vi "PC_AO to DCCM no trigger_Current.vi"() -> ()   [LabVIEW 2021]
uses:
  DC-RMS Current Measurement/Typedefs/Range and Terminal Settings.ctl
  DC-RMS Current Measurement/Typedefs/Specific Channel Settings.ctl
  DC-RMS Current Measurement/Typedefs/DC and RMS Current Measurements.ctl
  DC Voltage Generation/DAQ_DC Voltage Generation.lvlib
  DC-RMS Current Measurement/DAQ_DC-RMS Current Measurement.lvlib
panel:
  out "Current Waveforms":waveform(dbl)[](graph)=[{"t0"=timestamp(3825152084.7836895 s since 1904-01-01), "dt"=9.999999999999999e-05, "Y"=array[1000 elements], "attributes"=variant("NI_ChannelName"=variant(string "Dev1/ai2"), "NI_UnitDescription"=variant(string "Amps"))}, {"t0"=timestamp(3825152084.7837005 s since 1904-01-01), "dt"=9.999999999999999e-05, "Y"=array[1000 elements], "attributes"=variant("NI_ChannelName"=variant(string "Dev1/ai3"), "NI_UnitDescription"=variant(string "Amps"))}, {"t0"=timestamp(3825152084.7837114 s since 1904-01-01), "dt"=9.999999999999999e-05, "Y"=array[1000 elements], "attributes"=variant("NI_ChannelName"=variant(string "Dev1/ai4"), "NI_UnitDescription"=variant(string "Amps"))}]
  out "DC and RMS Current Measurements":T1={"Average DC Current (A)"=[0.0010007603119317984, 0.000998840528943941, 0.0004976560804234391], "RMS Current (A)"=[0.001000760315342945, 0.0009988405306055512, 0.0004976560812893033]} {"RMS Current (A)" format="%#.2p"; "Average DC Current (A)" format="%#.2p"}
  in  "Range and Terminal Settings":T2={"Global Settings"={"Min Range (A)"=-0.001, "Max Range (A)"=0.001, "Terminal Configuration"=10083, "Shunt Resistor (Ohm)"=1000.0}, "Specific Channel Settings"=[{"Active Channels"="Dev1/ai2", "Min Range"=-0.002, "Max Range"=0.002, "Terminal Configuration"=10106, "Shunt Resistor (ohms)"=5000.0}, {"Active Channels"="Dev1/ai3", "Min Range"=-0.002, "Max Range"=0.002, "Terminal Configuration"=10083, "Shunt Resistor (ohms)"=5000.0}, {"Active Channels"="Dev1/ai4", "Min Range"=-0.001, "Max Range"=0.001, "Terminal Configuration"=10083, "Shunt Resistor (ohms)"=10000.0}]} {"Specific Channel Settings"."Shunt Resistor (ohms)" format="%#.2p"; "Specific Channel Settings"."Terminal Configuration" items=["RSE"=10083, "NRSE"=10078, "Differential"=10106]; "Specific Channel Settings"."Max Range" format="%#.2p"; "Specific Channel Settings"."Min Range" format="%#.2p"; "Global Settings"."Shunt Resistor (Ohm)" format="%.2p"; "Global Settings"."Terminal Configuration" items=["RSE"=10083, "NRSE"=10078, "Differential"=10106]; "Global Settings"."Max Range (A)" format="%.2p"; "Global Settings"."Min Range (A)" format="%.2p"}
  out "error out":errorcluster
  # "Min. Range(A)"
  # "Max. Range(A)"
  # "Terminal Configuration"
  # "Shunt\nResistor(Ohm)"
  # "Physical Channel Name"
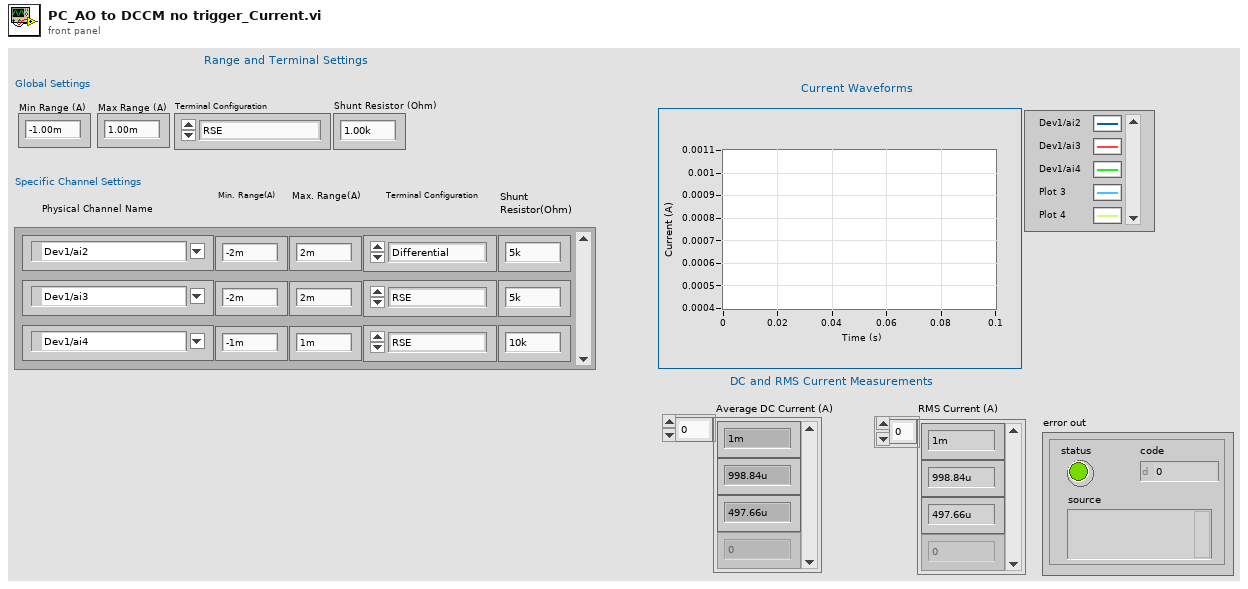
[diagram p1: front panel]
types:
  T1 = typedef "DAQ_DC-RMS Current Measurement.lvlib/DC and RMS Current Measurements.ctl" = cluster{"Average DC Current (A)":dbl[], "RMS Current (A)":dbl[]}
  T2 = typedef "DAQ_DC-RMS Current Measurement.lvlib/Range and Terminal Settings.ctl" = cluster{"Global Settings":cluster{"Min Range (A)":dbl, "Max Range (A)":dbl, "Terminal Configuration":i32, "Shunt Resistor (Ohm)":dbl}, "Specific Channel Settings":T3[]}
  T3 = typedef "DAQ_DC-RMS Current Measurement.lvlib/Specific Channel Settings.ctl" = cluster{"Active Channels":tag, "Min Range":dbl, "Max Range":dbl, "Terminal Configuration":i32, "Shunt Resistor (ohms)":dbl}
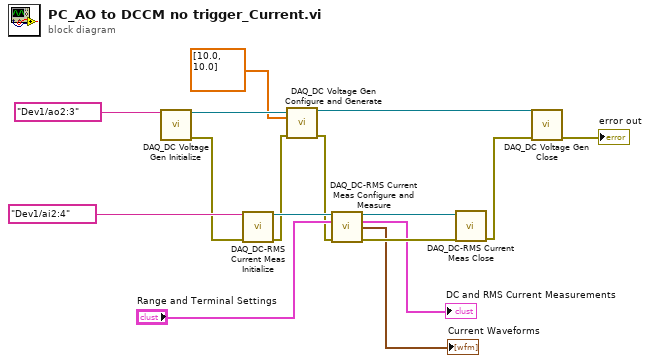
[diagram p0: block diagram]
diagram:
  n1 = call "DAQ_DC Voltage Gen Initialize.vi"("Physical Channels"=tag "Dev1/ao2:3") -> ("DAQmx Task Out"=w7:refnum<k21>, "error out"=w9:errorcluster)  [unwired: 13 in]
  n2 = call "DAQ_DC-RMS Current Meas Initialize.vi"("Physical Channels"=tag "Dev1/ai2:4", "error in"=w9) -> ("DAQmx Task Out"=w14:refnum<k21>, "error out"=w6:errorcluster)  [unwired: 12 in]
  n3 = call "DAQ_DC Voltage Gen Configure and Generate.vi"("DAQmx Task In"=w7, "Output Voltages (V)"=dbl[] [10.0, 10.0], "error in"=w6) -> ("DAQmx Task Out"=w3:refnum<k21>, "error out"=w5:errorcluster)  [unwired: 11 in]
  n4 = call "DAQ_DC-RMS Current Meas Configure and Measure.vi"("DAQmx Task In"=w14, "Range and Terminal Settings"="Range and Terminal Settings", "error in"=w5) -> ("DAQmx Task Out"=w16:refnum<k21>, "DC and RMS Current Measurements"=→"DC and RMS Current Measurements":T1, "Current Waveforms"=→"Current Waveforms":waveform(dbl)[], "error out"=w15:errorcluster)  [unwired: 8 in, 1 out]
  n5 = call "DAQ_DC-RMS Current Meas Close.vi"("DAQmx Task In"=w16, "error in"=w15) -> ("error out"=w4:errorcluster)  [unwired: 13 in]
  n6 = call "DAQ_DC Voltage Gen Close.vi"("DAQmx Task In"=w3, "error in"=w4) -> ("error out"=→"error out":errorcluster)  [unwired: 13 in]
